vi "Get value string.vi"(8 "error in (no error)":errorcluster, 11 "Column in":refnum<class "By-Value Column.lvclass">) -> (0 "error out":errorcluster, 2 "Value":string, 3 "Column out":refnum<class "By-Value Column.lvclass">)   [LabVIEW 2020, in "Basic Columns.lvlib" / "By-Value Column.lvclass"]
uses:
  By-Value Column.lvclass
  By-Value Column.lvclass/By-Value Column.ctl
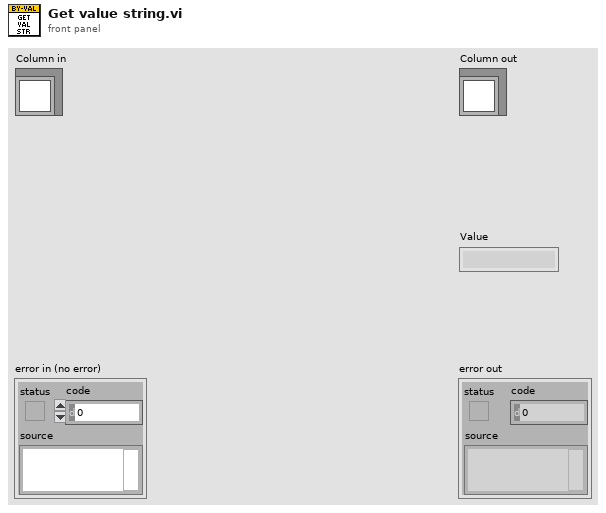
[diagram p1: front panel]
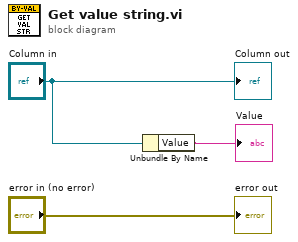
[diagram p0: block diagram]
diagram:
  n1 = Unbundle By Name("Column in") -> ("Value"=→"Value":string)
  "error out" <- "error in (no error)"
  "Column out" <- "Column in"
